vi "n select cor table.vi"(8 "error in (no error)":errorcluster, 9 "headb":u16, 10 "heada":u16, 11 "n":u16) -> (0 "error out":errorcluster)   [LabVIEW 2015, in "SCANalone4x64.lvlib"]
doc: "__declspec(dllimport) void __stdcall n_select_cor_table(unsigned short n, unsigned short heada, unsigned short headb);"
uses:
  <userlib>/SCANalone4x64/SCANalone4x64.lvlib
  <userlib>/SCANalone4x64/SCANalone4x64.dll
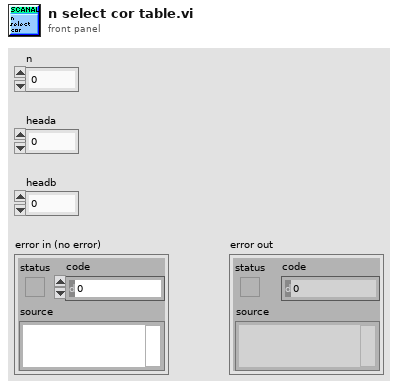
[diagram p1: front panel]
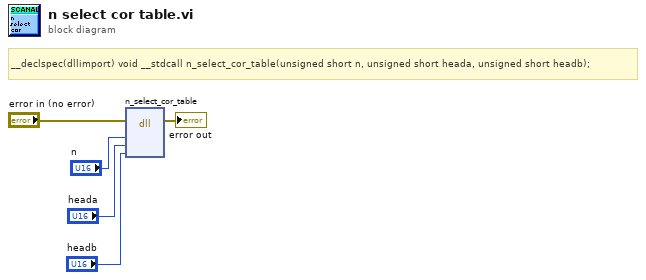
[diagram p0: block diagram]
diagram:
  # "__declspec(dllimport) void __stdcall n_select_cor_table(unsigned short n, unsigned short heada, unsigned short headb);"
  n1 = dll-call lib="C:/Program Files/National Instruments/LabVIEW 2015/user.lib/SCANalone4x64/SCANalone4x64.*" fn="n_select_cor_table"(error in="error in (no error)", "n"="n", "heada"="heada", "headb"="headb") -> (error out=→"error out":errorcluster)  [unwired: 6 in, 1 out]
